vi "Launch_HMI.vi"(8 "error in (no error)":errorcluster caption="entrée d'erreur (pas d'erreur)", 11 "Class Popup (Default) en entrée":refnum<class "Class Popup (Main).lvclass">) -> (0 "error out":errorcluster caption="sortie d'erreur", 3 "Class Popup (Default) en sortie":refnum<class "Class Popup (Main).lvclass">)   [LabVIEW 2020, in "Library Instrument & Equipement.lvlib" / "Library Popup.lvlib" / "Class Popup (Main).lvclass"]
uses:
  Class Popup (Main).lvclass
  Commun VI/TypeDef/Liste Error.ctl
  Class Popup (Main).lvclass/Class Popup (Main).ctl
  Commun VI/Library Commun.lvlib
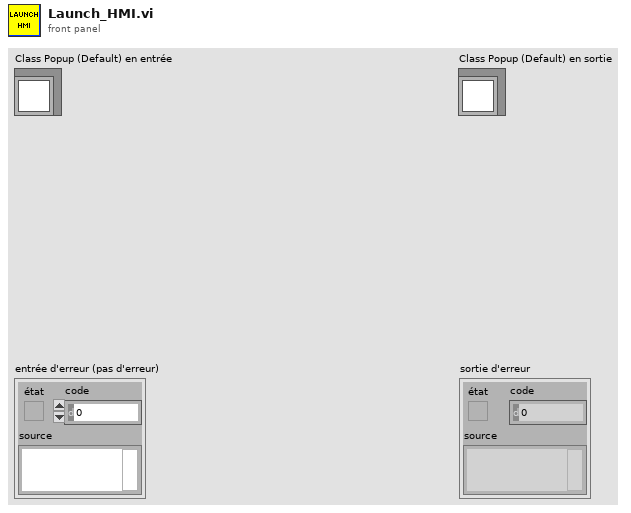
[diagram p1: front panel]
types:
  T1 = typedef "Library Commun.lvlib/Liste Error.ctl" = enum16{"Firebase Driver - Get Document", "Firebase Driver - Get Document With Where", "Firebase Driver - Delete Document", "Firebase Driver - Set Document", "Firebase Driver - Update Document", "Firebase Altyor - Search Document Bench", "Firebase Altyor - Class Not in Firebase", "Spectrum_Analyser - Timeout", "Relay Board - Qty Relay", "DIO - Pb Funtion", "Power_Supply - Peripherical not find", "Mutimeter - Peripherical not find", "Instrument - Function Not Used", "Instrument - Instrument name not specified", "Instrument - Allready Initialised", "Instrument - TimeOut", "Instrument - the instrument must be Initialise before", "Instrument - Frame Not received", "Instrument - Frame Nok", "Test - Initialise the File_for_Save", "Test - Timeout", "Test - Cmd Error", "FGV - Variable ", "BDD FireBase - Define Class", "SN - Class Not Define"}
  T2 = enum16{"Get Variable", "Get All Variables", "Set Variable", "Delete Variable", "Delete All Variable"}
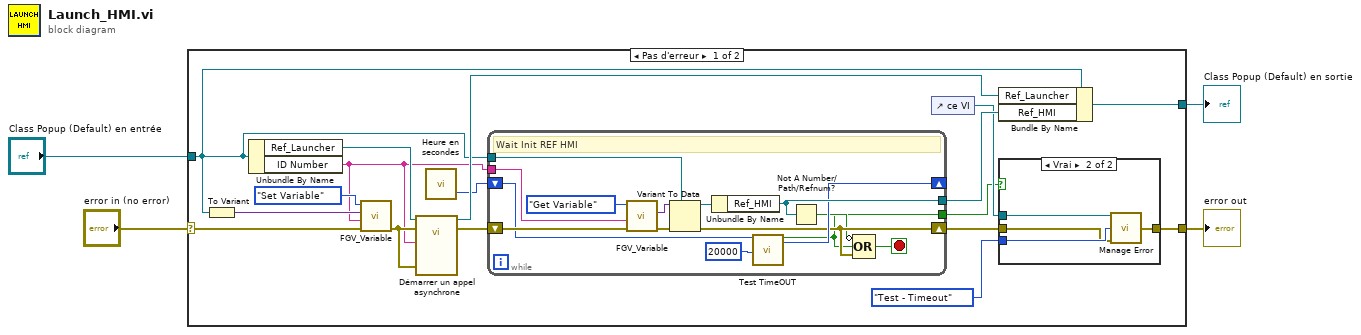
[diagram p0: block diagram]
diagram:
  n1 = case shown="Pas d'erreur" "error in (no error)" {
    selector: "error in (no error)" -> [w19 w43]
    tunnel: [w6 w43] -> w3
    tunnel: [w21 w42] -> w2
    tunnel: "Class Popup (Default) en entrée" -> [w14 w42]
    frame No Error {
      n2 = To Variant(anything=w14) -> (Variant=w16:variant)
      n3 = Unbundle By Name(w14) -> ("Ref_Launcher"=w13:refnum<vi>, "ID Number"=w12:string)
      n4 = call "FGV_Variable.vi"("error in (no error)"=w19, "Variable"=w12, "Data In"=w16, "Function"=T2."Set Variable") -> ("error out"=w18:errorcluster)  [unwired: 5 in, 2 out]
      n5 = call-by-ref "Démarrer un appel asynchrone"(reference=w13, error in=w18, 8:"error in (no error)"=w18, "ID"=w12) -> (reference out=w20:refnum<vi>, error out=w11:errorcluster)  [unwired: 7 in, 3 out]
      n6 = call "Heure en secondes.vi"() -> ("Heure en milisecondes"=w10:u32)  [unwired: 2 in, 1 out]
      n7 = while {
        tunnel: [w34] -> w15
        tunnel: w14 -> [w37]
        tunnel: w12 -> [w36]
        shift-right: [w29] -> w7
        shift-left: w11 -> [w35]
        shift-right: [w32] -> _
        shift-left: w10 -> [w33]
        tunnel: [w27] -> w5
        stop <- w31 stop-if-true
        # "Wait Init REF HMI"
        n8 = call "FGV_Variable.vi"("error in (no error)"=w35, "Variable"=w36, "Function"=T2."Get Variable") -> ("error out"=w40:errorcluster, "Data Out"=w39:variant)  [unwired: 6 in, 1 out]
        n9 = Variant To Data(error in=w40, type=w37, Variant=w39) -> (data=w38:refnum<class "Class Popup (Main).lvclass">, error out=w29:errorcluster)
        n10 = Unbundle By Name(w38) -> ("Ref_HMI"=w34:refnum<vi>)
        n11 = call "Test TimeOUT.vi"("OLD Time"=w33, "TimeOut ms"=u32 20000) -> ("Timeout ?"=w27:bool, "NEW Time"=w32:u32)  [unwired: 13 in, 3 out]
        n12 = Not A Number/Path/Refnum?(number/path/refnum=w34) -> (NaN/Path/Refnum?=w28:bool)
        n13 = Compound Arithmetic op=OR ("Opérateur arithmétique")(invert w28, w27, w29) -> (w31:bool)
      }
      n14 = control-ref of="ce VI"() -> (w8:refnum<vi>)
      n15 = Bundle By Name(cluster=w14, "Ref_Launcher"=w20, "Ref_HMI"=w15) -> (w21:refnum<class "Class Popup (Main).lvclass">)
      n16 = case shown="Vrai" w5 {
        tunnel: Liste_Error."Test - Timeout" ("Code Erreur") -> [_ w26]
        tunnel: w8 -> [_ w25]
        tunnel: w7 -> [w22 w24]
        tunnel: [w22 w23] -> w6
        frame False {
        }
        frame True {
          n17 = call "Manage Error.vi"("VI in Error"=w25, "Code Erreur"=w26, "error in (no error)"=w24) -> ("error out"=w23:errorcluster)  [unwired: 12 in]
        }
      }
    }
    frame Error {
    }
  }
  "error out" <- w3
  "Class Popup (Default) en sortie" <- w2
